vi "GetXL_CellValues_2D_String.vi"(8 "error in":errorcluster, 9 "End":cluster{"Column":i32, "Row":i32}, 10 "Start":cluster{"Column":i32, "Row":i32}, 11 "Refnum Cluster In":T1) -> (0 "error out":errorcluster, 2 "data":string[][](array[string]), 3 "Refnum Cluster Out":T1)   [LabVIEW 2017, in "excel_configuration.lvlib"]
uses:
  excel_configuration.lvlib
  0eea4b8d-c82f-4f8e-a307-16ae564bd13b.vi
  <vilib>/Utility/error.llb/Clear Errors.vi
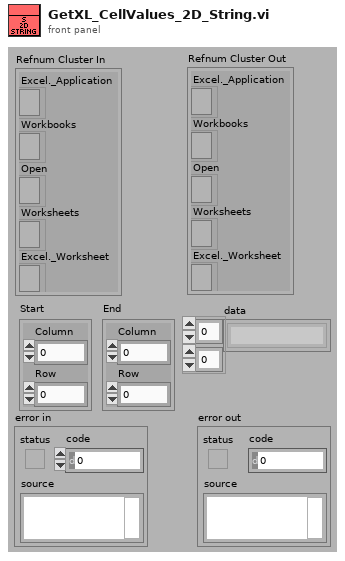
[diagram p1: front panel]
types:
  T1 = cluster{"Excel._Application":refnum<k7>, "Workbooks":refnum<k7>, "Open":refnum<k7>, "Worksheets":refnum<k7>, "Excel._Worksheet":refnum<k7>}
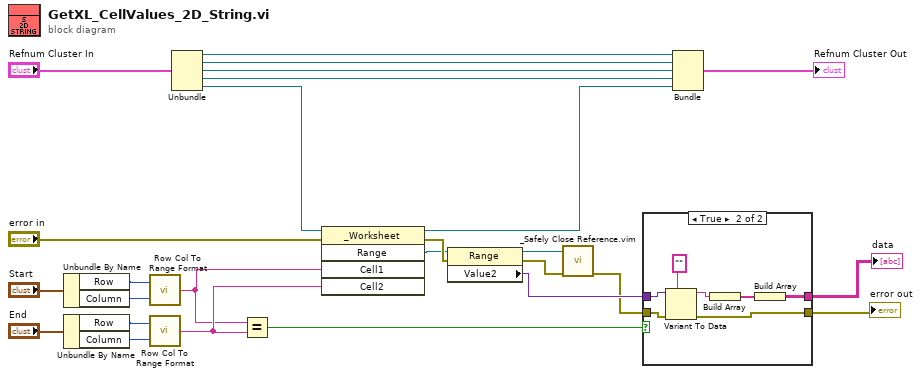
[diagram p0: block diagram]
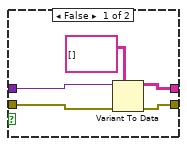
[diagram p2: hidden frame]
diagram:
  n1 = Unbundle By Name("Start") -> ("Row"=w12:i32, "Column"=w11:i32)
  n2 = Unbundle By Name("End") -> ("Row"=w9:i32, "Column"=w8:i32)
  n3 = call "Row Col To Range Format.vi"("Column"=w11, "Row"=w12) -> ("Output String"=w2:string)
  n4 = call "Row Col To Range Format.vi"("Column"=w8, "Row"=w9) -> ("Output String"=w3:string)
  n5 = Unbundle("Refnum Cluster In") -> ("Excel._Application"=w22:refnum<k7>, "Workbooks"=w23:refnum<k7>, "Open"=w24:refnum<k7>, "Worksheets"=w25:refnum<k7>, "Excel._Worksheet"=w21:refnum<k7>)
  n6 = Equal?(x=w2, y=w3) -> (x = y?=w1:bool)
  n7 = invoke class="_Worksheet" method="Range"(reference=w21, error in="error in", "Cell1"=w2, "Cell2"=w3) -> (reference out=w26:refnum<k7>, error out=w18:errorcluster, "Range"=w17:refnum<k7>)  [unwired: 1 in, 2 out]
  n8 = property class="Range"(reference=w17, error in=w18) -> (reference out=w15:refnum<k7>, error out=w14:errorcluster, "Value2"=w7:variant)
  n9 = call "_Safely Close Reference.vim"("error in (no error)"=w14, "Automation Refnum in"=w15) -> ("error out"=w6:errorcluster)  [unwired: 9 in]
  n10 = case shown="True" w1 {
    tunnel: w7 -> [w31 w37]
    tunnel: w6 -> [w30 w38]
    tunnel: [w29 w36] -> w5
    tunnel: [w27 w32] -> w4
    frame False {
      n11 = Variant To Data(error in=w30, type=string[][] [], Variant=w31) -> (data=w27:string[][], error out=w29:errorcluster)
    }
    frame True {
      n12 = Variant To Data(error in=w38, type="", Variant=w37) -> (data=w34:string, error out=w36:errorcluster)
      n13 = Build Array(w34) -> (w33:string[])
      n14 = Build Array(w33) -> (w32:string[][])
    }
  }
  "error out" <- w5
  "data" <- w4
  n15 = Bundle("Excel._Application"=w22, "Workbooks"=w23, "Open"=w24, "Worksheets"=w25, "Excel._Worksheet"=w26) -> (→"Refnum Cluster Out":T1)  [unwired: 1 in]
